vi "1.5.10.1-Number Generator.vi"() -> (0 "Number":u8)   [LabVIEW 2010]
doc: "Generates a new u8 each time it is called. u8s increment."
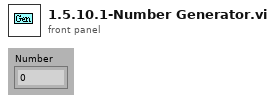
[diagram p1: front panel]
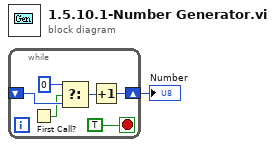
[diagram p0: block diagram]
diagram:
  n1 = while {
    shift-right: [w7] -> w1
    shift-left: _ -> [w4]
    stop <- TRUE stop-if-true
    n2 = First Call?() -> (First Call?: T/F=w3:bool)
    n3 = Select(t=u8 0, s=w3, f=w4) -> (s? t:f=w5:u8)
    n4 = Increment(x=w5) -> (x+1=w7:u8)
  }
  "Number" <- w1
